vi "SA5G_setupEVM.vi"(5 "SA_SCP_FILE":path=path "C:/TEMP/Demo/Distance Test/06_FR2_100M_120K_TDD_64QAM.wfm", 7 "max_dBm":i32, 8 "error in":errorcluster, 11 "VISA in":refnum<visa-resource-name>) -> (0 "error out":errorcluster, 2 "SA_Resp":string, 3 "VISA out":refnum<visa-resource-name>)   [LabVIEW 2020, in "Keysight.lvlib"]
uses:
  Keysight.lvlib
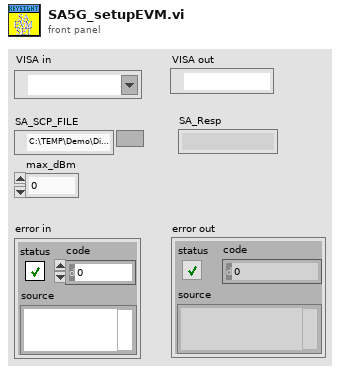
[diagram p1: front panel]
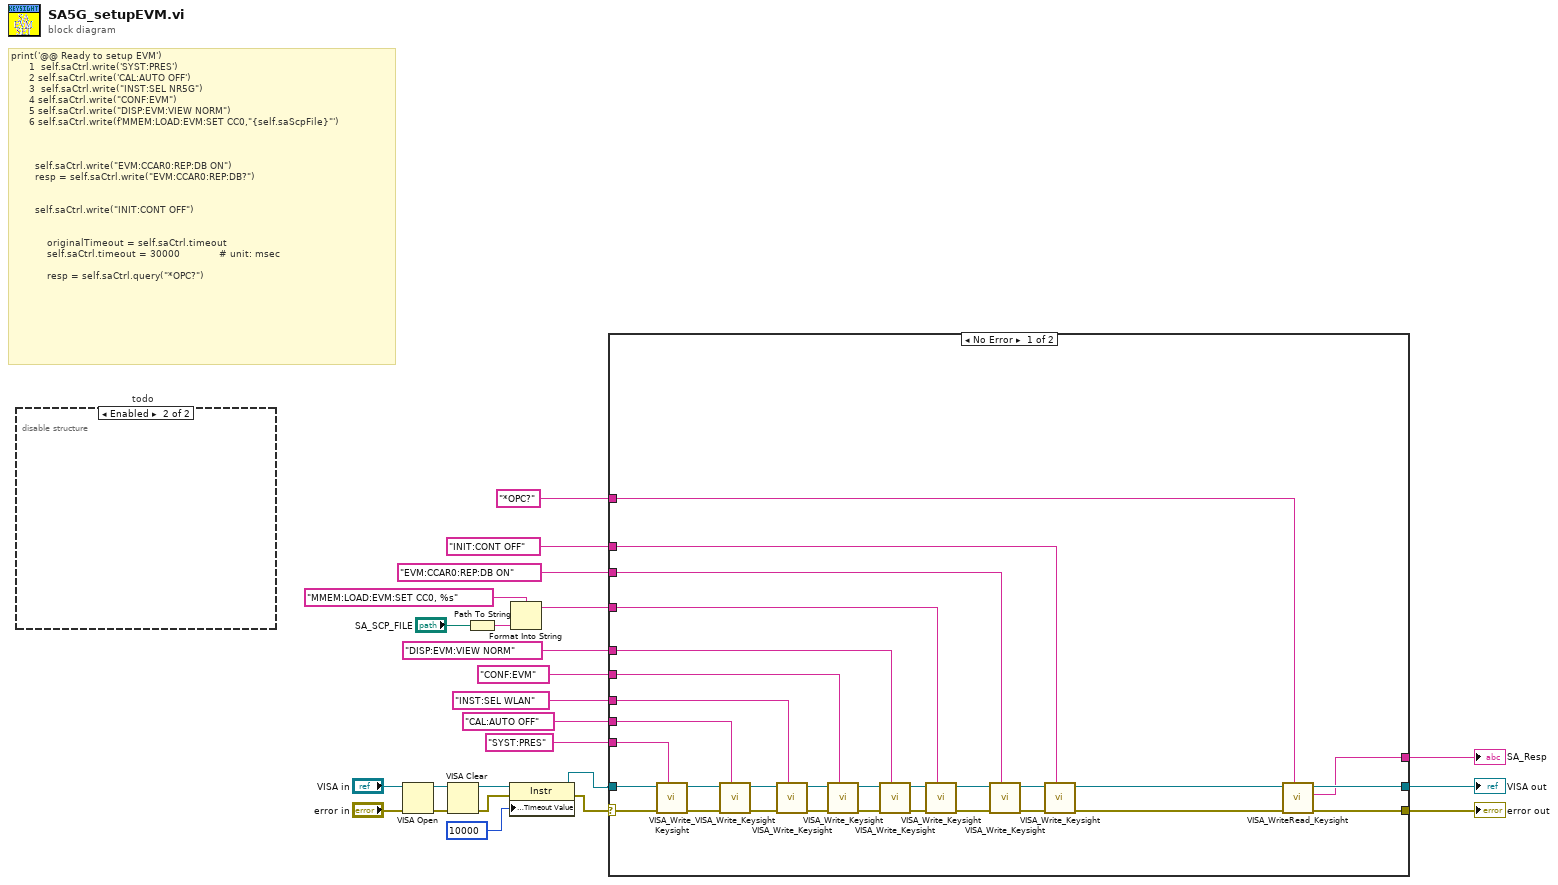
[diagram p0: block diagram]
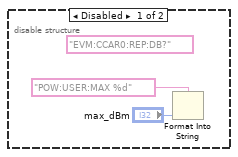
[diagram p2: hidden frame]
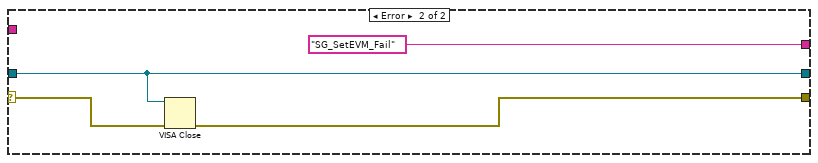
[diagram p3: hidden frame]
diagram:
  # "print('@@ Ready to setup EVM')\n      1  self.saCtrl.write('SYST:PRES')              \n      2 self.saCtrl.write('CAL:AUTO OFF')          \n      3  self.saCtrl.write(\"INST:SEL NR5G\")\n      4 self.saCtrl.write(\"CONF:EVM\")\n      5 self.saCtrl.write(\"DISP:EVM:VIEW NORM\")\n      6 self.saCtrl.write(f'MMEM:LOAD:EVM:SET CC0,\"{self.saScpFile}\"')\n\n        \n\n        self.saCtrl.write(\"EVM:CCAR0:REP:DB ON\")\n        resp = self.saCtrl.write(\"EVM:CCAR0:REP:DB?\")\n\n\n        self.saCtrl.write(\"INIT:CONT OFF\")\n\n\n            originalTimeout = self.saCtrl.timeout\n            self.saCtrl.timeout = 30000             # unit: msec\n\n            resp = self.saCtrl.query(\"*OPC?\")"
  n1 = disable-structure "todo" shown="Enabled" {
    frame Disabled {
      (unwired) "EVM:CCAR0:REP:DB?" ("write buffer")
      n2 = Format Into String(format string="POW:USER:MAX %d", "max_dBm") -> ()  [unwired: 2 in, 2 out]
    }
    frame Enabled {
    }
  }
  n3 = VISA Open(error in (no error)="error in", VISA resource name="VISA in") -> (VISA resource name=w7:refnum<visa-resource-name>, error out=w8:errorcluster)  [unwired: 3 in]
  n4 = VISA Clear(VISA resource name=w7, error in (no error)=w8) -> (VISA resource name out=w10:refnum<visa-resource-name>, error out=w9:errorcluster)
  n5 = Path To String(path="SA_SCP_FILE") -> (string=w19:string)
  n6 = property on="Property Node" class="Instr"(reference=w10, error in=w9, "General Settings:Timeout Value"=u32 10000) -> (reference out=w5:refnum<visa-resource-name>, error out=w6:errorcluster)
  n7 = Format Into String(format string="MMEM:LOAD:EVM:SET CC0, %s", w19) -> (resulting string=w2:string)  [unwired: 2 in, 1 out]
  n8 = case shown="No Error" w6 {
    selector: w6 -> [w56 w59]
    tunnel: w5 -> [w55 w57]
    tunnel: "SYST:PRES" ("write buffer") -> [w54 _]
    tunnel: "CAL:AUTO OFF" ("write buffer") -> [w51 _]
    tunnel: "INST:SEL WLAN" ("write buffer") -> [w48 _]
    tunnel: "CONF:EVM" ("write buffer") -> [w45 _]
    tunnel: "DISP:EVM:VIEW NORM" ("write buffer") -> [w42 _]
    tunnel: "EVM:CCAR0:REP:DB ON" ("write buffer") -> [w33 _]
    tunnel: "*OPC?" ("write buffer") -> [w28 _]
    tunnel: [w39 w58] -> w12
    tunnel: [w38 w57] -> w13
    tunnel: [w37 "SG_SetEVM_Fail" ("Response")] -> w14
    tunnel: w2 -> [w36 _]
    tunnel: "INIT:CONT OFF" ("write buffer") -> [w30 _]
    frame No Error {
      n9 = call "VISA_Write_Keysight.vi"("VISA CMD"=w54, "error in"=w56, "VISA in"=w55) -> ("error out"=w53:errorcluster, "VISA out"=w52:refnum<visa-resource-name>)  [unwired: 7 in]
      n10 = call "VISA_Write_Keysight.vi"("VISA CMD"=w51, "error in"=w53, "VISA in"=w52) -> ("error out"=w50:errorcluster, "VISA out"=w49:refnum<visa-resource-name>)  [unwired: 7 in]
      n11 = call "VISA_Write_Keysight.vi"("VISA CMD"=w48, "error in"=w50, "VISA in"=w49) -> ("error out"=w47:errorcluster, "VISA out"=w46:refnum<visa-resource-name>)  [unwired: 7 in]
      n12 = call "VISA_Write_Keysight.vi"("VISA CMD"=w45, "error in"=w47, "VISA in"=w46) -> ("error out"=w44:errorcluster, "VISA out"=w43:refnum<visa-resource-name>)  [unwired: 7 in]
      n13 = call "VISA_Write_Keysight.vi"("VISA CMD"=w42, "error in"=w44, "VISA in"=w43) -> ("error out"=w41:errorcluster, "VISA out"=w40:refnum<visa-resource-name>)  [unwired: 7 in]
      n14 = call "VISA_Write_Keysight.vi"("VISA CMD"=w36, "error in"=w41, "VISA in"=w40) -> ("error out"=w35:errorcluster, "VISA out"=w34:refnum<visa-resource-name>)  [unwired: 7 in]
      n15 = call "VISA_Write_Keysight.vi"("VISA CMD"=w33, "error in"=w35, "VISA in"=w34) -> ("error out"=w32:errorcluster, "VISA out"=w29:refnum<visa-resource-name>)  [unwired: 7 in]
      n16 = call "VISA_Write_Keysight.vi"("VISA CMD"=w30, "error in"=w32, "VISA in"=w29) -> ("error out"=w31:errorcluster, "VISA out"=w27:refnum<visa-resource-name>)  [unwired: 7 in]
      n17 = call "VISA_WriteRead_Keysight.vi"("VISA_CMD"=w28, "error in"=w31, "VISA in"=w27) -> ("error out"=w39:errorcluster, "Response"=w37:string, "VISA out"=w38:refnum<visa-resource-name>)  [unwired: 6 in]
    }
    frame Error {
      n18 = VISA Close(VISA resource name=w57, error in (no error)=w59) -> (error out=w58:errorcluster)
    }
  }
  "SA_Resp" <- w14
  "VISA out" <- w13
  "error out" <- w12
